vi "Update_Event_Statistics.vi"(7 "Total_coincidence_time":dbl, 8 "Status/Errors in":refnum<vi>, 9 "Page Statistics 2":refnum<vi>, 10 "Event statistics":T1[](array[typedef]), 11 "Page Statistics":refnum<vi>) -> (0 "Status/Errors out":refnum<vi>)   [LabVIEW 2013]
uses:
  Controls/Event_Statistics.ctl
  Controls/Get_Set_Statistics_Options.ctl
  Controls/Fill_Histogram_Options.ctl
  Controls/Get_Set_Statistics_Options2.ctl
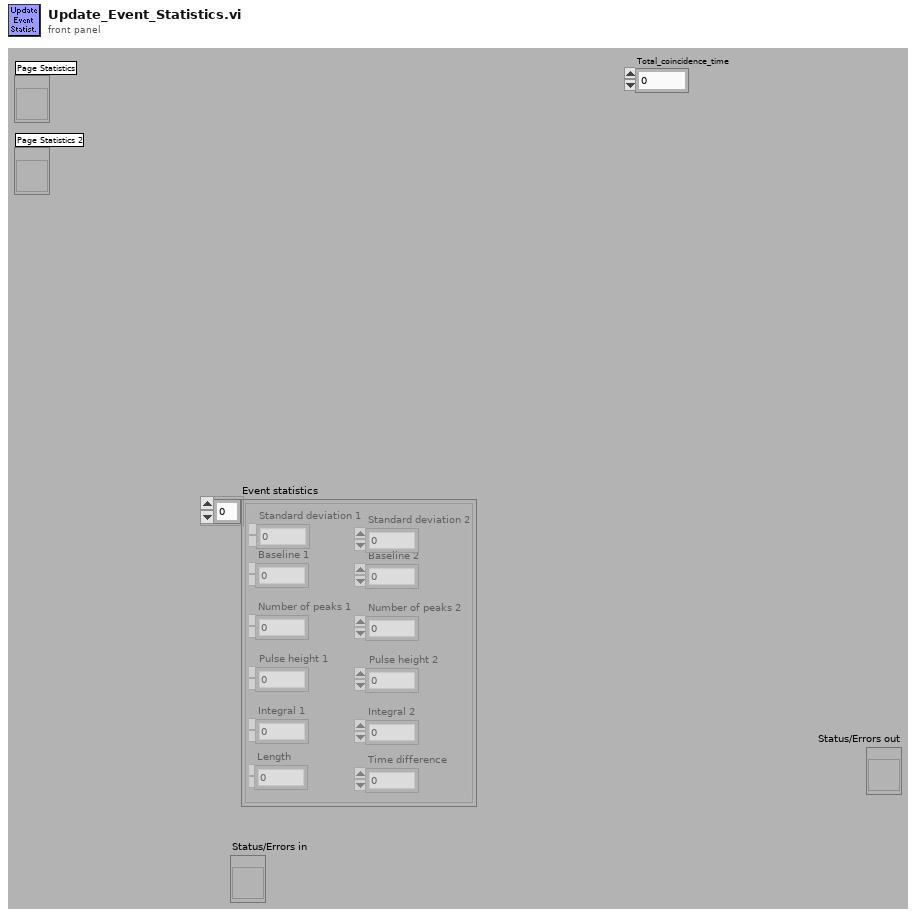
[diagram p1: front panel]
types:
  T1 = typedef "Event_Statistics.ctl" = cluster{"Baseline 1":i16, "Baseline 2":i16, "Number of peaks 1":i16, "Number of peaks 2":i16, "Pulse height 1":i16, "Pulse height 2":i16, "Integral 1":i32, "Integral 2":i32, "Standard deviation 1":i16, "Standard deviation 2":i16, "Length":i32, "Time difference":u32}
  T2 = typedef "Fill_Histogram_Options.ctl" = enum16{"Number of peaks", "Pulse height", "Integral", "Baseline", "Standard deviation", "Time difference", "Time difference 2", "Length"}
  T3 = typedef "Get_Set_Statistics_Options2.ctl" = enum16{"Get", "Set"}
  T4 = typedef "Get_Set_Statistics_Options.ctl" = enum16{"Get", "Set singles", "Set events"}
  T5 = typedef "TabPage_Statistics2.ctl" = cluster{"Baseline_overshoot":dbl, "St.Dev.overshoot":dbl, "Data points overshoot":dbl, "Time difference overshoot":dbl, "Time_difference_zoom_count":dbl, "Baseline.His":cluster{"t0":i32, "dt":i32, "Histogram":i32[][]}, "St._dev.His":cluster{"t0":i32, "dt":i32, "Histogram":i32[][]}, "Trace_length.His":cluster{"t0":i32, "dt":i32, "Histogram":i32[][]}, "Time_difference.His_zoom":cluster{"t0":i32, "dt":i32, "Histogram":i32[][]}, "Time_difference.His":cluster{"t0":i32, "dt":i32, "Histogram":i32[][]}, "Baselin Entries":u64, "Baseline Overshoots":u64, "Time Entries ":u64, "Time  Overshoots ":u64, "St.dev. Entries ":u64, "St.dev.  Overshoots ":u64, "Length  Entries ":u64, "Length Overshoots ":u64, "Time zoom Entries ":u64, "Time zoom Overshoots ":u64}
  T6 = typedef "TabPage_Statistics.ctl" = cluster{"Thresh_Count_MAS":T7, "Thresh_Count_SLV":T7, "Count":bool, "Time_to_count":u32, "Time":u32, "Time_to_count_ref":refnum<vi>, "Counting?":bool, "Baseline_MAS_Ch1":i16, "Baseline_MAS_Ch2":i16, "Baseline_SLV_Ch1":i16, "Baseline_SLV_Ch2":i16, "Basel_Err_MAS_Ch1":u32, "Basel_Err_MAS_Ch2":u32, "Basel_Err_SLV_Ch1":u32, "Basel_Err_SLV_Ch2":u32, "Peaks_Overshoot":dbl, "Height_Overshoot":dbl, "Integrals_Overshoot":dbl, "Last_event":dbl, "Total_Trigger":u32, "Av_Trigger":dbl, "Number of peaks":cluster{"t0":i32, "dt":i32, "Histogram":i32[][]}, "Pulse height":cluster{"t0":i32, "dt":i32, "Histogram":i32[][]}, "Integral":cluster{"t0":i32, "dt":i32, "Histogram":i32[][]}, "Number of peaks Entries":u64, "Number of peaks Overshoots":u64, "Pulse height  Entries":u64, "Pulse height Overshoots":u64, "Integral Entries":u64, "Integral Overshoots":u64, "Last trigger Stack":refnum<vi>}
  T7 = typedef "Page_Thresholds.ctl" = cluster{"Sing_Ch1_low":u32, "Sing_Ch1_high":u32, "Sing_Ch2_low":u32, "Sing_Ch2_high":u32, "Total_Ch1_low":u32, "Total_Ch1_high":u32, "Total_Ch2_low":u32, "Total_Ch2_high":u32, "Av_Ch1_low":dbl, "Av_Ch1_high":dbl, "Av_Ch2_low":dbl, "Av_Ch2_high":dbl}
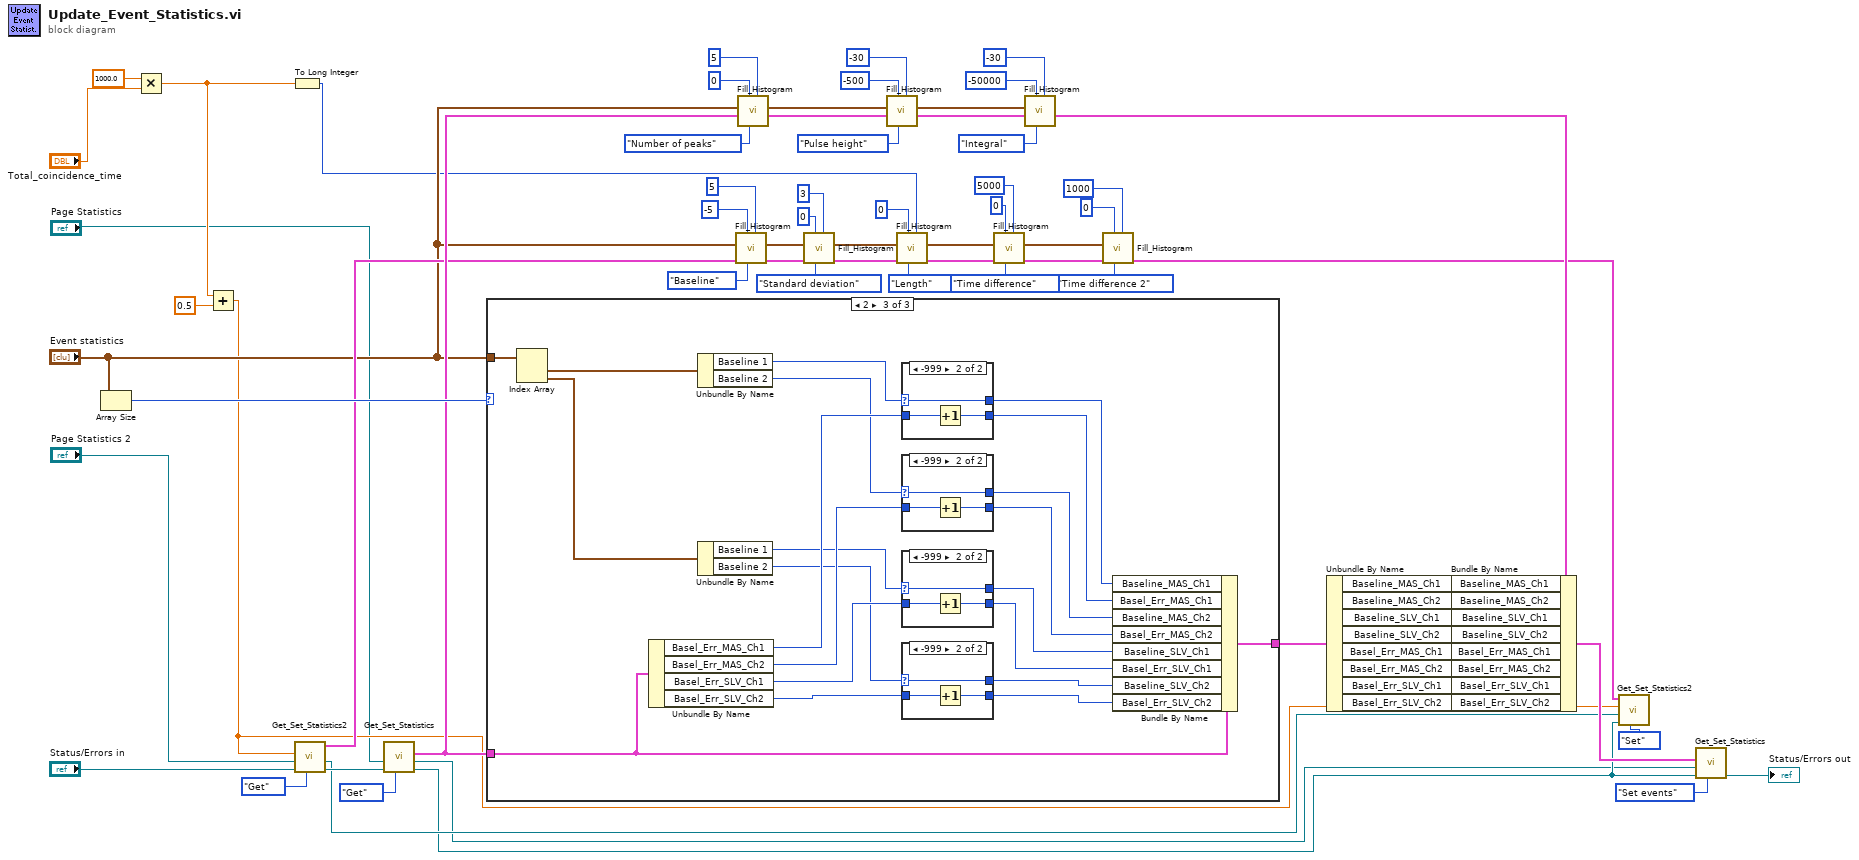
[diagram p0: block diagram]
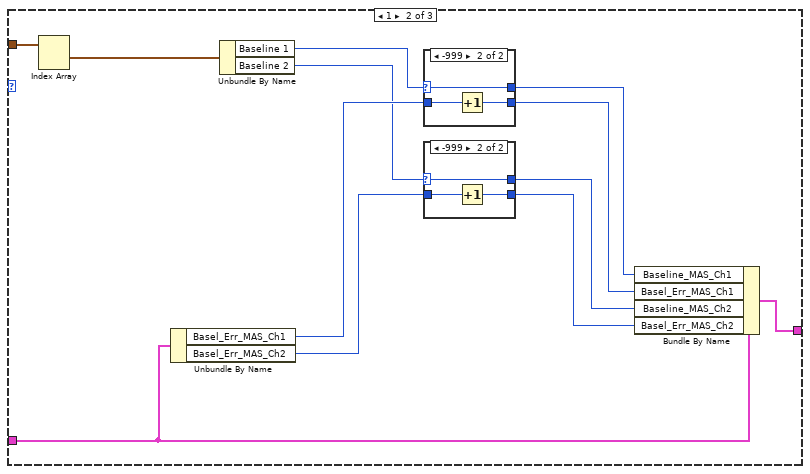
[diagram p3: hidden frame]
diagram:
  n1 = Array Size(array="Event statistics") -> (size(s)=w66:i32)
  n2 = Multiply(x=1000.0, y="Total_coincidence_time") -> (x*y=w5:dbl)
  n3 = Add(x=w5, y=0.5) -> (x+y=w3:dbl)
  n4 = To Long Integer(number=w5) -> (32bit integer=w6:i32)
  n5 = call "Get_Set_Statistics2.vi"("Get/Set"=Get_Set_Statistics_Options2."Get", "Status/Errors in"="Status/Errors in", "Page Statistics 2"="Page Statistics 2", "Time window"=w3) -> ("Status/Errors out"=w40:refnum<vi>, "Page Statistics 2"=w11:refnum<vi>, "Page Statistics 2 out"=w38:T5)  [unwired: 1 in, 4 out]
  n6 = call "Get_Set_Statistics.vi"("Page Statistics in"="Page Statistics", "Status/Errors in"=w40, "Get/Set"=Get_Set_Statistics_Options."Get") -> ("Value out"=w65:T6, "Page Statistics out"=w1:refnum<vi>, "Status/Errors out"=w9:refnum<vi>)  [unwired: 1 in, 4 out]
  n7 = case shown="2" w66 {
    tunnel: w65 -> [w70 w79 w109]
    tunnel: [w70 w82 w113] -> w57
    tunnel: "Event statistics" -> [_ w81 w112]
    frame Default {
    }
    frame 1 {
      n8 = Index Array(array=w81) -> (element #1=w80:T1)  [unwired: 2 in, 1 out]
      n9 = Unbundle By Name(w79) -> ("Basel_Err_MAS_Ch1"=w78:u32, "Basel_Err_MAS_Ch2"=w73:u32)
      n10 = Unbundle By Name(w80) -> ("Baseline 1"=w76:i16, "Baseline 2"=w74:i16)
      n11 = case shown="-999" w76 {
        selector: w76 -> [w88 w90]
        tunnel: w78 -> [w89 w92]
        tunnel: [w89 w91] -> w77
        tunnel: [w88 w90] -> w75
        frame Default {
        }
        frame -999 {
          n12 = Increment(x=w92) -> (x+1=w91:u32)
        }
      }
      n13 = case shown="-999" w74 {
        selector: w74 -> [w83 w85]
        tunnel: w73 -> [w84 w87]
        tunnel: [w84 w86] -> w71
        tunnel: [w83 w85] -> w72
        frame Default {
        }
        frame -999 {
          n14 = Increment(x=w87) -> (x+1=w86:u32)
        }
      }
      n15 = Bundle By Name(cluster=w79, "Baseline_MAS_Ch1"=w75, "Basel_Err_MAS_Ch1"=w77, "Baseline_MAS_Ch2"=w72, "Basel_Err_MAS_Ch2"=w71) -> (w82:T6)
    }
    frame 2 {
      n16 = Index Array(array=w112) -> (element #1=w111:T1, element #2=w110:T1)  [unwired: 2 in]
      n17 = Unbundle By Name(w109) -> ("Basel_Err_MAS_Ch1"=w108:u32, "Basel_Err_MAS_Ch2"=w103:u32, "Basel_Err_SLV_Ch1"=w102:u32, "Basel_Err_SLV_Ch2"=w95:u32)
      n18 = Unbundle By Name(w111) -> ("Baseline 1"=w106:i16, "Baseline 2"=w104:i16)
      n19 = Unbundle By Name(w110) -> ("Baseline 1"=w101:i16, "Baseline 2"=w96:i16)
      n20 = case shown="-999" w106 {
        selector: w106 -> [w129 w131]
        tunnel: w108 -> [w130 w133]
        tunnel: [w130 w132] -> w107
        tunnel: [w129 w131] -> w105
        frame Default {
        }
        frame -999 {
          n21 = Increment(x=w133) -> (x+1=w132:u32)
        }
      }
      n22 = case shown="-999" w104 {
        selector: w104 -> [w124 w126]
        tunnel: w103 -> [w125 w128]
        tunnel: [w125 w127] -> w99
        tunnel: [w124 w126] -> w100
        frame Default {
        }
        frame -999 {
          n23 = Increment(x=w128) -> (x+1=w127:u32)
        }
      }
      n24 = case shown="-999" w101 {
        selector: w101 -> [w119 w121]
        tunnel: w102 -> [w120 w123]
        tunnel: [w120 w122] -> w97
        tunnel: [w119 w121] -> w98
        frame Default {
        }
        frame -999 {
          n25 = Increment(x=w123) -> (x+1=w122:u32)
        }
      }
      n26 = case shown="-999" w96 {
        selector: w96 -> [w114 w116]
        tunnel: w95 -> [w115 w118]
        tunnel: [w115 w117] -> w93
        tunnel: [w114 w116] -> w94
        frame Default {
        }
        frame -999 {
          n27 = Increment(x=w118) -> (x+1=w117:u32)
        }
      }
      n28 = Bundle By Name(cluster=w109, "Baseline_MAS_Ch1"=w105, "Basel_Err_MAS_Ch1"=w107, "Baseline_MAS_Ch2"=w100, "Basel_Err_MAS_Ch2"=w99, "Baseline_SLV_Ch1"=w98, "Basel_Err_SLV_Ch1"=w97, "Baseline_SLV_Ch2"=w94, "Basel_Err_SLV_Ch2"=w93) -> (w113:T6)
    }
  }
  n29 = call "Fill_Histogram.vi"("Maximum"=5 ("Minimum"), "Histogram 2"=Fill_Histogram_Options."Baseline" ("Histogram"), "Minimum"=-5, "Page statistics 2 in"=w38, "Event statistics in"="Event statistics") -> ("Page statistics 2 out"=w37:T5, "Event statistics out"=w36:T1[])  [unwired: 2 in, 3 out]
  n30 = call "Fill_Histogram.vi"("Maximum"=5 ("Minimum"), "Histogram 2"=Fill_Histogram_Options."Number of peaks" ("Histogram"), "Minimum"=0, "Page Statistics in"=w65, "Event statistics in"="Event statistics") -> ("Page Statistics out"=w61:T6, "Event statistics out"=w59:T1[])  [unwired: 2 in, 3 out]
  n31 = call "Fill_Histogram.vi"("Maximum"=3 ("Minimum"), "Histogram 2"=Fill_Histogram_Options."Standard deviation" ("Histogram"), "Minimum"=0, "Page statistics 2 in"=w37, "Event statistics in"=w36) -> ("Page statistics 2 out"=w26:T5, "Event statistics out"=w24:T1[])  [unwired: 2 in, 3 out]
  n32 = call "Fill_Histogram.vi"("Maximum"=-30 ("Minimum"), "Histogram 2"=Fill_Histogram_Options."Pulse height" ("Histogram"), "Minimum"=-500, "Page Statistics in"=w61, "Event statistics in"=w59) -> ("Page Statistics out"=w60:T6, "Event statistics out"=w58:T1[])  [unwired: 2 in, 3 out]
  n33 = call "Fill_Histogram.vi"("Maximum"=w6, "Histogram 2"=Fill_Histogram_Options."Length" ("Histogram"), "Minimum"=0, "Page statistics 2 in"=w26, "Event statistics in"=w24) -> ("Page statistics 2 out"=w21:T5, "Event statistics out"=w22:T1[])  [unwired: 2 in, 3 out]
  n34 = call "Fill_Histogram.vi"("Maximum"=5000, "Histogram 2"=Fill_Histogram_Options."Time difference" ("Histogram"), "Minimum"=0, "Page statistics 2 in"=w21, "Event statistics in"=w22) -> ("Page statistics 2 out"=w13:T5, "Event statistics out"=w17:T1[])  [unwired: 2 in, 3 out]
  n35 = call "Fill_Histogram.vi"("Maximum"=-30 ("Minimum"), "Histogram 2"=Fill_Histogram_Options."Integral" ("Histogram"), "Minimum"=-50000, "Page Statistics in"=w60, "Event statistics in"=w58) -> ("Page Statistics out"=w56:T6)  [unwired: 2 in, 4 out]
  n36 = call "Fill_Histogram.vi"("Maximum"=1000, "Histogram 2"=Fill_Histogram_Options."Time difference 2" ("Histogram"), "Minimum"=0, "Page statistics 2 in"=w13, "Event statistics in"=w17) -> ("Page statistics 2 out"=w12:T5)  [unwired: 2 in, 4 out]
  n37 = Unbundle By Name(w57) -> ("Baseline_MAS_Ch1"=w55:i16, "Baseline_MAS_Ch2"=w54:i16, "Baseline_SLV_Ch1"=w53:i16, "Baseline_SLV_Ch2"=w52:i16, "Basel_Err_MAS_Ch1"=w51:u32, "Basel_Err_MAS_Ch2"=w50:u32, "Basel_Err_SLV_Ch1"=w49:u32, "Basel_Err_SLV_Ch2"=w48:u32)
  n38 = Bundle By Name(cluster=w56, "Baseline_MAS_Ch1"=w55, "Baseline_MAS_Ch2"=w54, "Baseline_SLV_Ch1"=w53, "Baseline_SLV_Ch2"=w52, "Basel_Err_MAS_Ch1"=w51, "Basel_Err_MAS_Ch2"=w50, "Basel_Err_SLV_Ch1"=w49, "Basel_Err_SLV_Ch2"=w48) -> (w47:T6)
  n39 = call "Get_Set_Statistics2.vi"("Get/Set"=Get_Set_Statistics_Options2."Set", "Status/Errors in"=w9, "Page Statistics 2"=w11, "Time window"=w3, "Page Statistics 2 in"=w12) -> ()  [unwired: 7 out]
  n40 = call "Get_Set_Statistics.vi"("Value in"=w47, "Page Statistics in"=w1, "Status/Errors in"=w9, "Get/Set"=Get_Set_Statistics_Options."Set events") -> ("Status/Errors out"=→"Status/Errors out":refnum<vi>)  [unwired: 6 out]
